vi "String - Unicode String to Hex String.vi"(11 "Unicode String in":string) -> (3 "Hex String out":string)   [LabVIEW 2020]
panel:
  # "bìN/f°e RaWlQlÿ\n\n?a\nNRÍyÏe0í0[Yeÿ\n\nâVÓ~Nôÿ\n\nú^¾lQcks^I{vl;N>yOÿ\n\nv^:N[°sýV¶[KNx^y0A~cNÛekÿ\n\nqQTªRR0"
  # "0x1162EC4E2F66B065A05261576C51116C0CFF0D000A00938A3F610D4E0652CD79CF650130008AED8B0130975B59650CFF0D000A00E256D37E004EF4810CFF0D000A00FA5EBE8B6C51636B735E497B8476116C3B4E3E791A4F0CFF0D000A00765E3A4E9E5BB073FD56B65B4B4E785E8F790130417E63830E4EDB8F656B0CFF0D000A0071510C54AA529B520230"
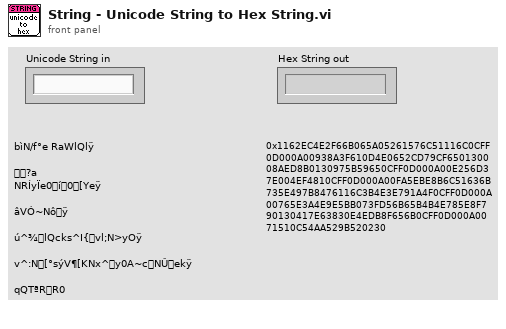
[diagram p1: front panel]
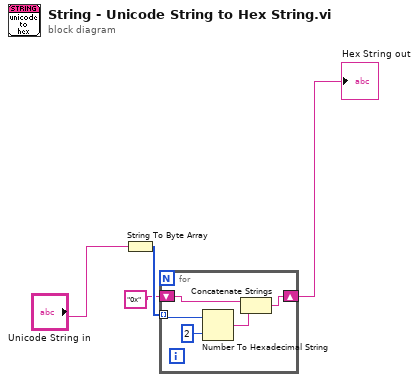
[diagram p0: block diagram]
diagram:
  n1 = String To Byte Array(string="Unicode String in") -> (unsigned byte array=w4:u8[])
  n2 = for {
    tunnel: w4 -> [w9] mode=indexing
    shift-right: [w7] -> w2
    shift-left: "0x" -> [w6]
    n3 = Number To Hexadecimal String(1:i16 2 ("width (-)"), 2:w9) -> (0:w8:string)
    n4 = Concatenate Strings(w6, w8) -> (w7:string)
  }
  "Hex String out" <- w2
